vi "Init.vi"(8 "error in (no error)":errorcluster, 11 "VISA resource in":refnum<visa-resource-name>) -> (0 "error out":errorcluster, 3 "VISA resource out":refnum<visa-resource-name>)   [LabVIEW 2020, in "Rename to match project.lvlib"]
uses:
  Rename to match project.lvlib
  Typedefs/Init.vi States.ctl
panel:
  in  "Connect Btn":bool
  # "1. VISA Resource/Comm Port"
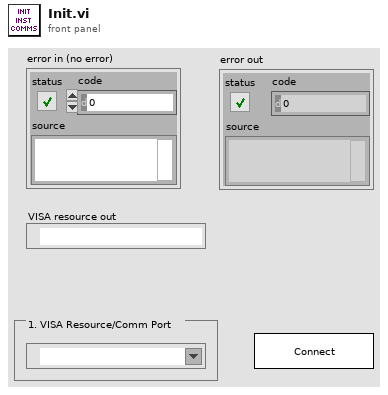
[diagram p1: front panel]
types:
  T1 = typedef "Rename to match project.lvlib/Init.vi States.ctl" = enum16{"Waiting for connection", "Connecting", "Successful connection", "Failed to connect", "Closing"}
  T2 = enum32{"Invalid", "Standard", "Closed", "Hidden", "Minimized", "Maximized"}
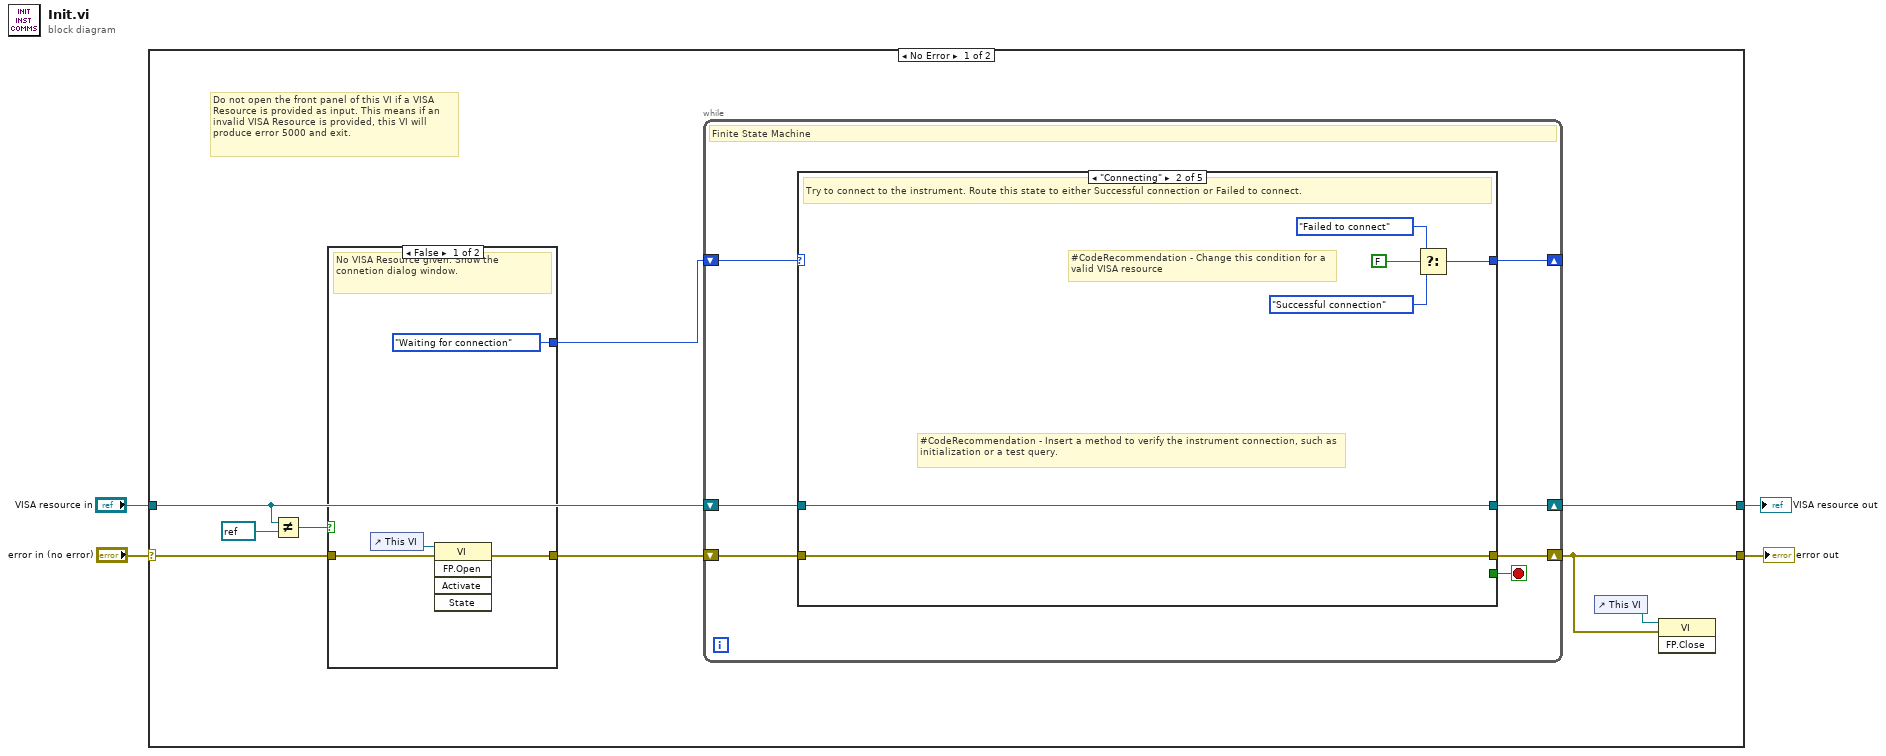
[diagram p0: block diagram]
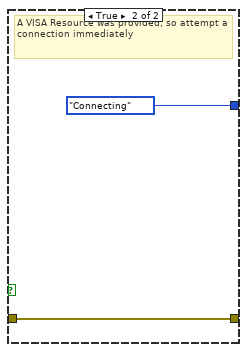
[diagram p2: hidden frame]
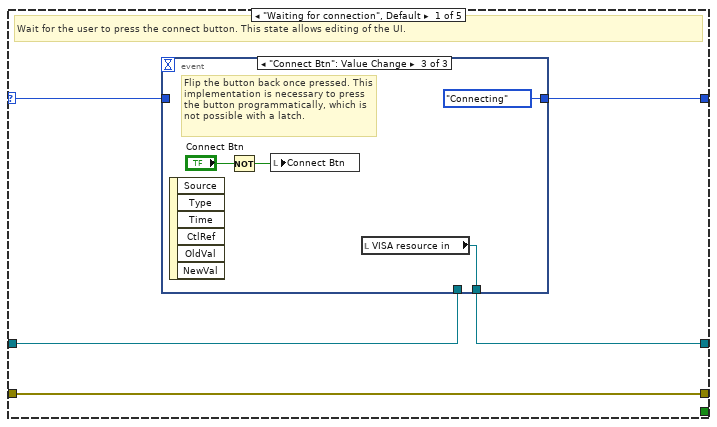
[diagram p3: hidden frame]
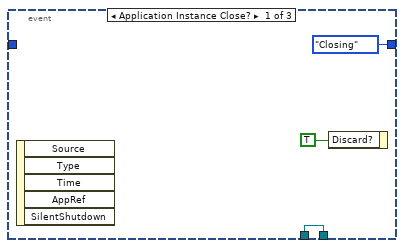
[diagram p4: hidden frame]
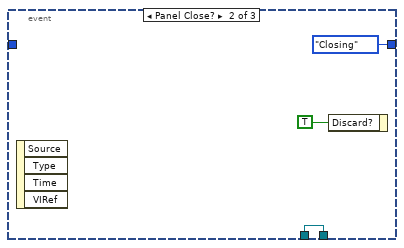
[diagram p5: hidden frame]
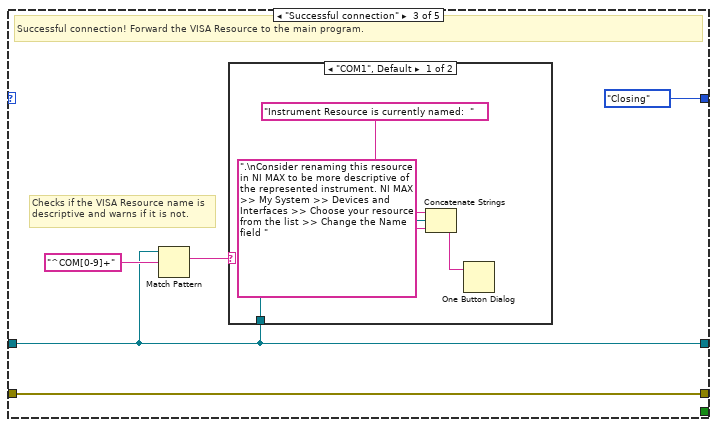
[diagram p6: hidden frame]
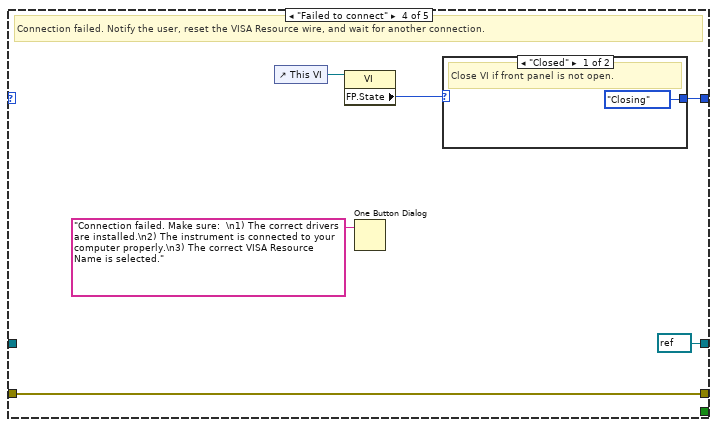
[diagram p8: hidden frame]
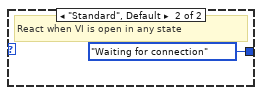
[diagram p9: hidden frame]
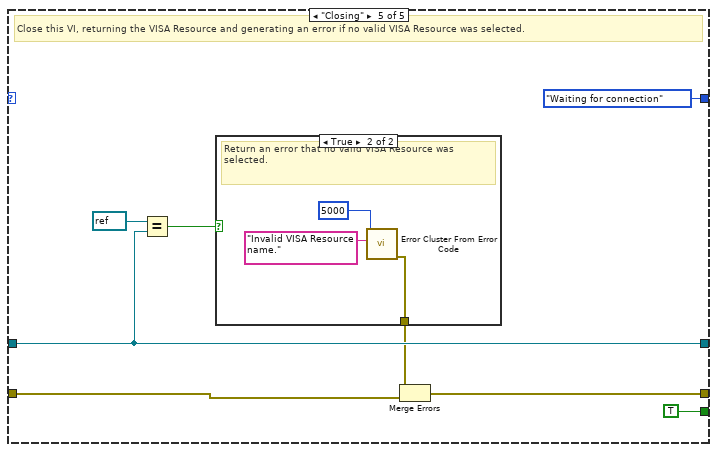
[diagram p10: hidden frame]
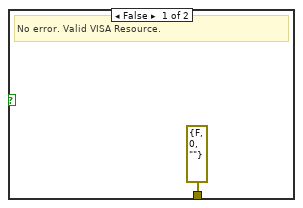
[diagram p11: hidden frame]
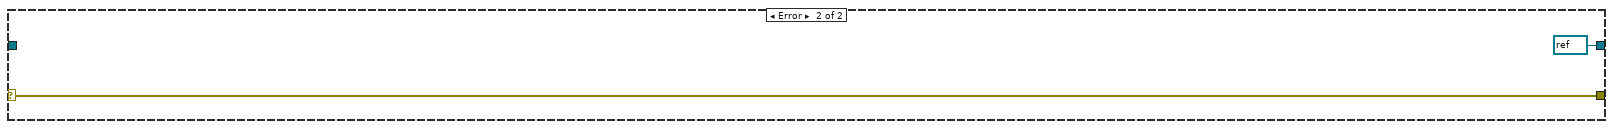
[diagram p12: hidden frame]
diagram:
  n1 = case shown="No Error" "error in (no error)" {
    selector: "error in (no error)" -> [w7 w78]
    tunnel: [w13 refnum<visa-resource-name> refnum ("VISA resource in")] -> w4
    tunnel: [w11 w78] -> w2
    tunnel: "VISA resource in" -> [w8 _]
    frame No Error {
      # "Do not open the front panel of this VI if a VISA Resource is provided as input. This means if an invalid VISA Resource is provided, this VI will produce error 5000 and exit."
      n2 = Not Equal?(x=w8, y=refnum<visa-resource-name> refnum ("x")) -> (x != y?=w10:bool)
      n3 = case shown="False" w10 {
        tunnel: w7 -> [w16 w19]
        tunnel: [w15 w19] -> w6
        tunnel: [Init.vi_States."Waiting for connection" Init.vi_States."Connecting"] -> w5
        frame False {
          # "No VISA Resource given. Show the connetion dialog window."
          n4 = control-ref of="This VI"() -> (w17:refnum<vi>)
          n5 = invoke class="VI" method="FP.Open"(reference=w17, error in=w16) -> (error out=w15:errorcluster)  [unwired: 3 in, 4 out]
        }
        frame True {
          # "A VISA Resource was provided, so attempt a connection immediately"
        }
      }
      n6 = while {
        shift-right: [w25] -> _
        shift-left: w5 -> [w26]
        shift-right: [w23] -> w13
        shift-left: w8 -> [w22]
        shift-right: [w20] -> w11
        shift-left: w6 -> [w21]
        stop <- w24 stop-if-true
        # "Finite State Machine"
        n7 = case shown="\"Connecting\"" w26 {
          selector: w26 -> [w31 _ _ _ _]
          tunnel: [w30 w47 Init.vi_States."Closing" w62 Init.vi_States."Waiting for connection"] -> w25
          tunnel: [_ _ _ _ TRUE] -> w24
          tunnel: [w28 w43 w48 refnum<visa-resource-name> refnum ("VISA resource in") w69] -> w23
          tunnel: w22 -> [w27 w43 w48 _ w69]
          tunnel: w21 -> [w29 w44 w51 w59 w65]
          tunnel: [w29 w44 w51 w59 w66] -> w20
          frame "Waiting for connection", Default {
            # "Wait for the user to press the connect button. This state allows editing of the UI."
            n8 = event shown="[2] \"Connect Btn\": Value Change" {
              selector: _ -> [_ _ _]
              dyn-events: _ -> [_ _ _]
              timeout: _ -> [_ _ _]
              tunnel: [Init.vi_States."Closing" Init.vi_States."Closing" Init.vi_States."Connecting"] -> w30
              tunnel: w31 -> [_ _ _]
              tunnel: [w32 w35 w38] -> w28
              tunnel: w27 -> [w32 w35 _]
              event Application Instance Close? {
                n9 = event-data() -> ()  [unwired: 1 in, 5 out]
                n10 = event-data("Discard?"=TRUE) -> ()  [unwired: 1 in, 1 out]
              }
              event Panel Close? {
                n11 = event-data() -> ()  [unwired: 1 in, 4 out]
                n12 = event-data("Discard?"=TRUE) -> ()  [unwired: 1 in, 1 out]
              }
              event "Connect Btn": Value Change {
                # "Flip the button back once pressed. This implementation is necessary to press the button programmatically, which is not possible with a latch."
                n13 = event-data() -> ()  [unwired: 1 in, 6 out]
                n14 = Not(x="Connect Btn") -> (.not. x?=w39:bool)
                n15 = local write "Connect Btn"(w39) -> ()
                n16 = local read "VISA resource in"() -> (w38:refnum<visa-resource-name>)
              }
            }
          }
          frame "Connecting" {
            # "#CodeRecommendation - Change this condition for a valid VISA resource"
            # "#CodeRecommendation - Insert a method to verify the instrument connection, such as initialization or a test query."
            # "Try to connect to the instrument. Route this state to either Successful connection or Failed to connect."
            n17 = Select(t=Init.vi_States."Failed to connect", s=FALSE, f=Init.vi_States."Successful connection") -> (s? t:f=w47:T1)
          }
          frame "Successful connection" {
            # "Checks if the VISA Resource name is descriptive and warns if it is not."
            # "Successful connection! Forward the VISA Resource to the main program."
            n18 = Match Pattern(string=w48, regular expression="^COM[0-9]+") -> (match substring=w49:string)  [unwired: 1 in, 3 out]
            n19 = case shown="\"COM1\", Default" w49 {
              tunnel: w48 -> [w54 _]
              frame "COM1", Default {
                n20 = Concatenate Strings("Instrument Resource is currently named:  ", w54, ".\nConsider renaming this resource in NI MAX to be more descriptive of the represented instrument. NI MAX >> My System >> Devices and Interfaces >> Choose your resource from the list >> Change the Name field " ("string")) -> (w56:string)
                n21 = One Button Dialog(message=w56) -> ()  [unwired: 1 in, 1 out]
              }
              frame "" {
              }
            }
          }
          frame "Failed to connect" {
            # "Connection failed. Notify the user, reset the VISA Resource wire, and wait for another connection."
            n22 = control-ref of="This VI"() -> (w58:refnum<vi>)
            n23 = property class="VI"(reference=w58) -> ("FP.State"=w57:T2)  [unwired: 1 in, 2 out]
            n24 = One Button Dialog(message="Connection failed. Make sure:  \n1) The correct drivers are installed.\n2) The instrument is connected to your computer properly.\n3) The correct VISA Resource Name is selected.") -> ()  [unwired: 1 in, 1 out]
            n25 = case shown="\"Closed\"" w57 {
              tunnel: [Init.vi_States."Closing" Init.vi_States."Waiting for connection"] -> w62
              frame "Closed" {
                # "Close VI if front panel is not open."
              }
              frame "Standard", Default {
                # "React when VI is open in any state"
              }
            }
          }
          frame "Closing" {
            # "Close this VI, returning the VISA Resource and generating an error if no valid VISA Resource was selected."
            n26 = Equal?(x=refnum<visa-resource-name> refnum ("VISA resource in"), y=w69) -> (x = y?=w68:bool)
            n27 = case shown="True" w68 {
              tunnel: [errorcluster {"status"=FALSE, "code"=0, "source"=""} ("error out") w75] -> w67
              frame False {
                # "No error. Valid VISA Resource."
              }
              frame True {
                # "Return an error that no valid VISA Resource was selected."
                n28 = call <vilib>:"Error Cluster From Error Code.vi"("error message (\"\")"="Invalid VISA Resource name." ("error message (\"\")"), "error code (0)"=5000) -> ("error out"=w75:errorcluster)  [unwired: 7 in]
              }
            }
            n29 = Merge Errors(w67, w65) -> (w66:errorcluster)
          }
        }
      }
      n30 = control-ref of="This VI"() -> (w12:refnum<vi>)
      n31 = invoke class="VI" method="FP.Close"(reference=w12, error in=w11) -> ()  [unwired: 1 in, 3 out]
    }
    frame Error {
    }
  }
  "VISA resource out" <- w4
  "error out" <- w2
